vi "Planning.vi"() -> ()   [LabVIEW 2015]
panel:
  out "Gap Sample Widths":dbl[](array[numeric])=[5000.0, 2948.610387317338, 1738.8606432391405, 1025.444510950448, 604.7272673212075, 356.6210203834683, 210.3072890076806, 124.02285137931928, 73.13901356835504, 43.13169102515907, 25.43571043586922, 15.0]
  out "Boxcar Sample Widths - Gaps":dbl[](array[numeric])=[1500.0, 1500.0, 1500.0, 1500.0, 1500.0, 1500.0, 1023.2157972085035, 506.7364263932681, 249.3983357054377, 121.79706284736254, 58.90023985078198, 28.125000000000007]
  out "All Detection Time Widths":dbl[](array[numeric])=[0.0013800000000000002, 0.0007056599208015297, 0.000360837625960595, 0.00018451351489678658, 9.435057413686829e-05, 4.82459555601459e-05, 2.467046172432368e-05, 1.2615185555451748e-05, 6.450746985475854e-06, 3.2985750774504324e-06, 1.686719005733024e-06, 8.625000000000001e-07]
  out "Boxcar Widths - Gaps":dbl[](array[numeric])=[3e-05, 3e-05, 3e-05, 3e-05, 3e-05, 3e-05, 2.046431594417007e-05, 1.0134728527865362e-05, 4.987966714108754e-06, 2.435941256947251e-06, 1.1780047970156395e-06, 5.625000000000001e-07]
  out "Gap Ratio":dbl=1.695714029057948
  out "Evenly Spaced Gaps":dbl[](array[numeric])=[0.0001, 5.897220774634676e-05, 3.477721286478281e-05, 2.0508890219008956e-05, 1.209454534642415e-05, 7.132420407669366e-06, 4.206145780153612e-06, 2.4804570275863855e-06, 1.4627802713671008e-06, 8.626338205031814e-07, 5.087142087173844e-07, 3e-07]
  out "Max Size Samples":dbl=3e-05
  out "Min Size Samples":dbl=1e-06
  out "Max Gap Samples":dbl=0.0001
  out "Min Gap Samples":dbl=3e-07
  in  "Max Size":dbl=3e-05
  in  "Min Size":dbl=1e-06
  in  "Max Gap":dbl=0.0001
  in  "Min Gap":dbl=3e-07
  out "Ratio":dbl=1.9556162385310416
  in  "No. of Filters":i32=11
  out "All Detection Sample Widths":dbl[](array[numeric])=[69000.00000000001, 35282.99604007648, 18041.88129802975, 9225.67574483933, 4717.5287068434145, 2412.297778007295, 1233.523086216184, 630.7592777725874, 322.5373492737927, 164.92875387252164, 84.3359502866512, 43.12500000000001]
  out "Evenly Spaced Particle Velocities":dbl[](array[numeric])=[100.0, 195.56162385310415, 382.4434872406299, 747.912693968215, 1462.6302093277388, 2860.343388327382, 5593.733977987928, 10939.197001376033, 21392.871292381053, 41836.24648818494, 81815.64299148167, 160000.0]
  in  "Clock Speed":dbl=50000000.0
  in  "PSU dist":dbl=1.62
  in  "PSU Width":dbl=0.2413
  in  "Detector dist":dbl=0.6
  in  "Detector width":dbl=0.138
  in  "Slowest particle":dbl=100.0
  in  "Fastest particle":dbl=160000.0
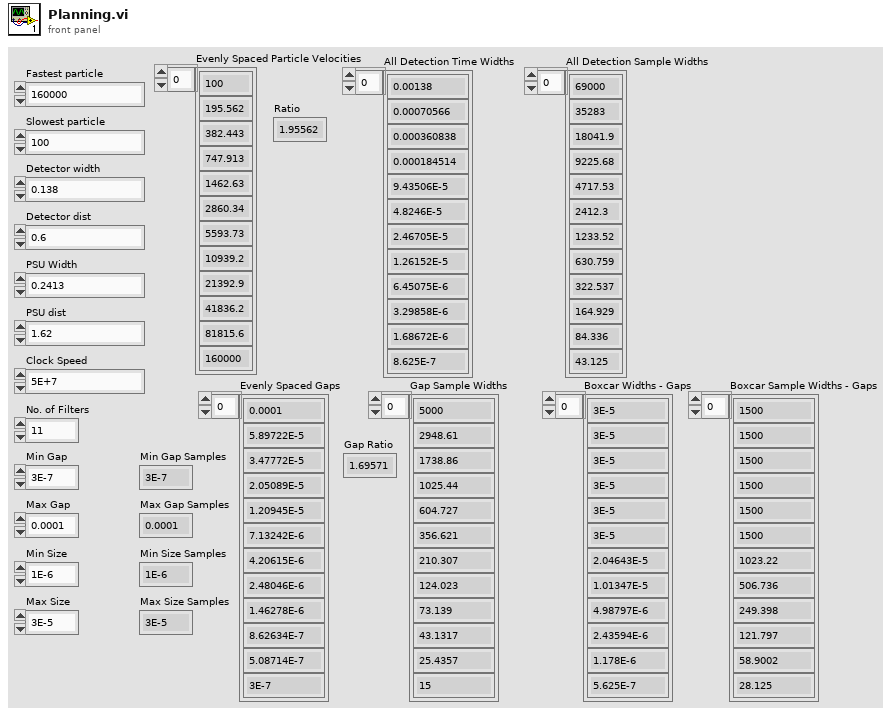
[diagram p1: front panel]
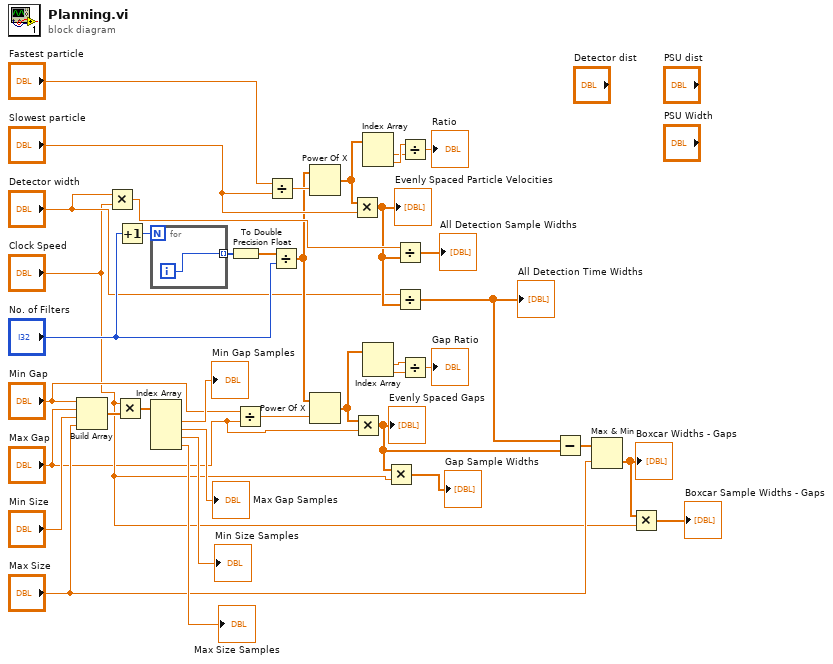
[diagram p0: block diagram]
diagram:
  n1 = Build Array("Min Gap", "Max Gap", "Min Size", "Max Size") -> (w25:dbl[])
  n2 = Multiply(x="Detector width", y="Clock Speed") -> (x*y=w33:dbl)
  n3 = Multiply(x="Clock Speed", y=w25) -> (x*y=w24:dbl[])
  n4 = Increment(x="No. of Filters") -> (x+1=w32:i32)
  n5 = for {
    N: w32 -> [_]
    tunnel: [w39] -> w36 mode=indexing
    i -> [w39]
  }
  n6 = Index Array(array=w24) -> (element #1=→"Min Gap Samples":dbl, element #2=→"Max Gap Samples":dbl, element #3=→"Min Size Samples":dbl, element #4=→"Max Size Samples":dbl)  [unwired: 4 in]
  n7 = To Double Precision Float(number=w36) -> (double precision float=w35:dbl[])
  n8 = Divide(x="Min Gap", y="Max Gap") -> (x/y=w21:dbl)
  n9 = Divide(x="Fastest particle", y="Slowest particle") -> (x/y=w34:dbl)
  n10 = Divide(x=w35, y="No. of Filters") -> (x/y=w20:dbl[])
  n11 = Power Of X(1:w34, 2:w20) -> (0:w30:dbl[])
  n12 = Power Of X(1:w21, 2:w20) -> (0:w15:dbl[])
  n13 = Multiply(x=w30, y="Slowest particle") -> (x*y=w13:dbl[])
  "Evenly Spaced Particle Velocities" <- w13
  n14 = Multiply(x=w15, y="Max Gap") -> (x*y=w3:dbl[])
  "Evenly Spaced Gaps" <- w3
  n15 = Index Array(array=w30) -> (element #1=w28:dbl, element #2=w29:dbl)  [unwired: 2 in]
  n16 = Index Array(array=w15) -> (element #1=w17:dbl, element #2=w16:dbl)  [unwired: 2 in]
  n17 = Multiply(x=w3, y="Clock Speed") -> (x*y=→"Gap Sample Widths":dbl[])
  n18 = Divide(x=w33, y=w13) -> (x/y=→"All Detection Sample Widths":dbl[])
  n19 = Divide(x="Detector width", y=w13) -> (x/y=w10:dbl[])
  "All Detection Time Widths" <- w10
  n20 = Divide(x=w29, y=w28) -> (x/y=→"Ratio":dbl)
  n21 = Divide(x=w17, y=w16) -> (x/y=→"Gap Ratio":dbl)
  n22 = Subtract(x=w10, y=w3) -> (x-y=w9:dbl[])
  n23 = Max & Min(x=w9, y="Max Size") -> (min(x,y)=w6:dbl[])  [unwired: 1 out]
  "Boxcar Widths - Gaps" <- w6
  n24 = Multiply(x=w6, y="Clock Speed") -> (x*y=→"Boxcar Sample Widths - Gaps":dbl[])
